vi "Framework.Create.Cache.vi"(8 "error in (no error)":errorcluster, 11 "Framework in":refnum<class "Framework.lvclass">) -> (0 "error out":errorcluster, 3 "Framework out":refnum<class "Framework.lvclass">)   [LabVIEW 2017, in "DSF Core.lvlib" / "Framework.lvclass"]
uses:
  Framework.lvclass
  Transfer/Transfer Group.lvclass
  Transfer/Transfer.lvclass
  Framework.lvclass/Framework.ctl
  Cache/Cache.lvclass
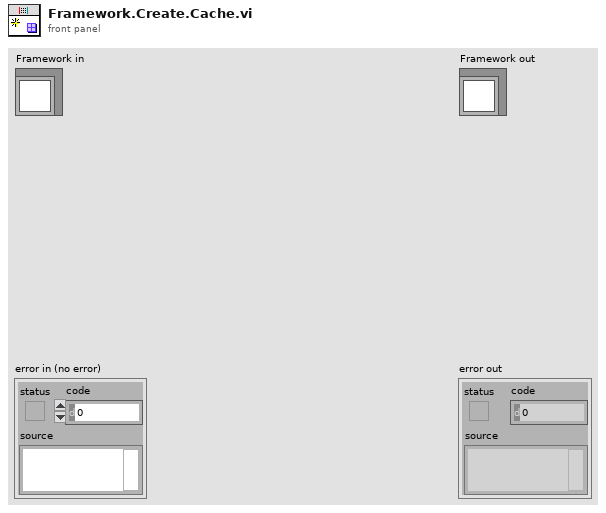
[diagram p1: front panel]
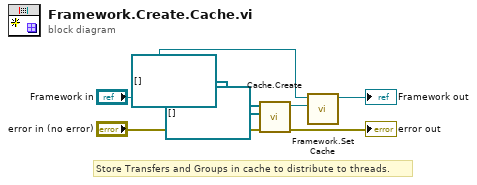
[diagram p0: block diagram]
diagram:
  # "Store Transfers and Groups in cache to distribute to threads."
  n1 = call "Cache.Create.vi"("error in (no error)"="error in (no error)", "Transfers"=refnum<class "Transfer.lvclass">[] [], "Transfers Groups"=refnum<class "Transfer Group.lvclass">[] []) -> ("error out"=→"error out":errorcluster, "Cache out"=w7:refnum<class "Cache.lvclass">)  [unwired: 7 in]
  n2 = call "Framework.Set Cache.vi"("Cache"=w7, "Framework in"="Framework in") -> ("Framework out"=→"Framework out":refnum<class "Framework.lvclass">)  [unwired: 9 in]
